vi "Mimetypes整体图.vi"() -> ()   [LabVIEW 2014]
panel:
  in  "Calculator":bool
  in  "Calc":bool
  in  "Calc template":bool
  in  "Build":bool
  in  "Bookcase":bool
  in  "Binary":bool
  in  "Audio":bool
  in  "Ascii":bool
  in  "Application":bool
  in  "Writer":bool
  in  "Writer template":bool
  in  "Wordprocessing":bool
  in  "Wine":bool
  in  "Widget_doc":bool
  in  "Video":bool
  in  "Vectorgfx":bool
  in  "Vcard":bool
  in  "Vcalendar":bool
  in  "Unknown":bool
  in  "Type":bool
  in  "Txt":bool
  in  "True type":bool
  in  "Track":bool
  in  "Tgz":bool
  in  "Text":bool
  in  "Tex":bool
  in  "Temp":bool
  in  "Temp (2)":bool
  in  "Tar":bool
  in  "Spreadsheet":bool
  in  "Sound":bool
  in  "Soffice":bool
  in  "Sign":bool
  in  "Shellscript":bool
  in  "Rpm":bool
  in  "Resource":bool
  in  "Recycled":bool
  in  "Record":bool
  in  "Real":bool
  in  "Real document":bool
  in  "Readme":bool
  in  "Quicktime":bool
  in  "Presenter":bool
  in  "Postscript":bool
  in  "Pens":bool
  in  "Pdf":bool
  in  "Patch":bool
  in  "Oo setup":bool
  in  "Netscape":bool
  in  "Multiple":bool
  in  "Mozilla":bool
  in  "Modeler":bool
  in  "Mime":bool
  in  "Midi":bool
  in  "Metafont":bool
  in  "Message":bool
  in  "Make":bool
  in  "Lyx":bool
  in  "Log":bool
  in  "Locked":bool
  in  "Lock":bool
  in  "Kword":bool
  in  "Kugardata":bool
  in  "Kugar":bool
  in  "Koffice":bool
  in  "Koffice (2)":bool
  in  "Kivio_flw":bool
  in  "Karbon":bool
  in  "Java":bool
  in  "Install":bool
  in  "Info":bool
  in  "Impress":bool
  in  "Impress template":bool
  in  "Image":bool
  in  "Html":bool
  in  "Help":bool
  in  "Gnome":bool
  in  "Gimp image":bool
  in  "Gf":bool
  in  "Get list":bool
  in  "Formula":bool
  in  "Font":bool
  in  "Font bitmap":bool
  in  "Encrypted":bool
  in  "Empty":bool
  in  "Empty (3)":bool
  in  "Empty (2)":bool
  in  "Ebuild":bool
  in  "Dvi":bool
  in  "Draw":bool
  in  "Draw template":bool
  in  "Draw (2)":bool
  in  "Document":bool
  in  "Doc":bool
  in  "Deb":bool
  in  "Corel":bool
  in  "Core":bool
  in  "Colorset":bool
  in  "Color":bool
  in  "Chart":bool
  in  "Cd list":bool
  in  "Cd image":bool
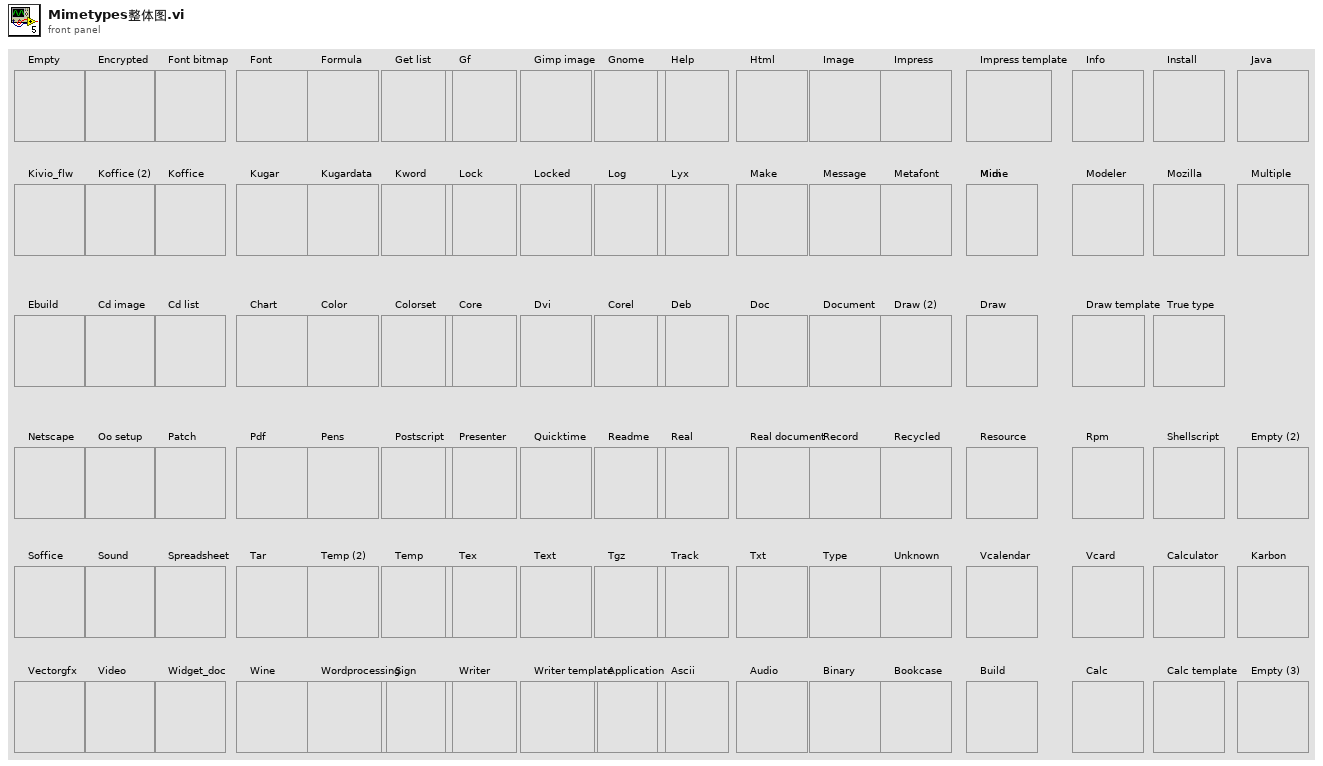
[diagram p1: front panel]
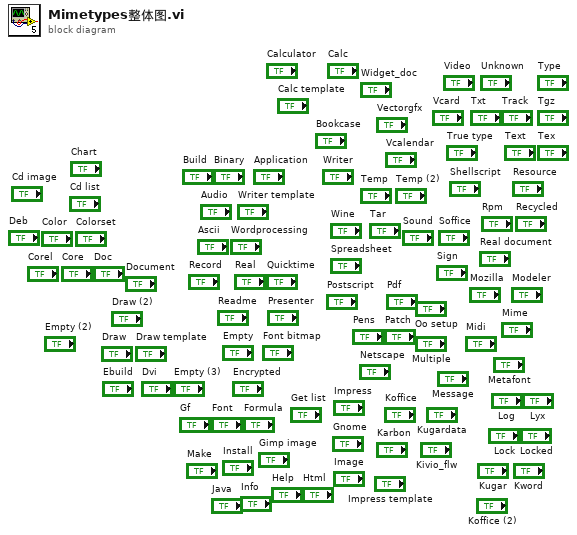
[diagram p0: block diagram]
diagram:
